vi "testMatOper.vi"(8 "error in (no error)":errorcluster) -> (0 "error out":errorcluster)   [LabVIEW 2016]
doc: "Test the MatOper class functions."
uses:
  <vilib>/addons/_JKI Toolkits/Caraya/classes/Test/Test.lvclass
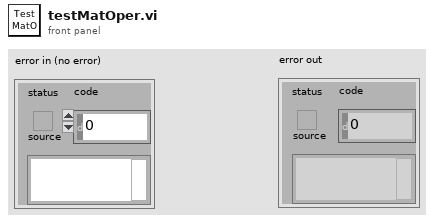
[diagram p1: front panel]
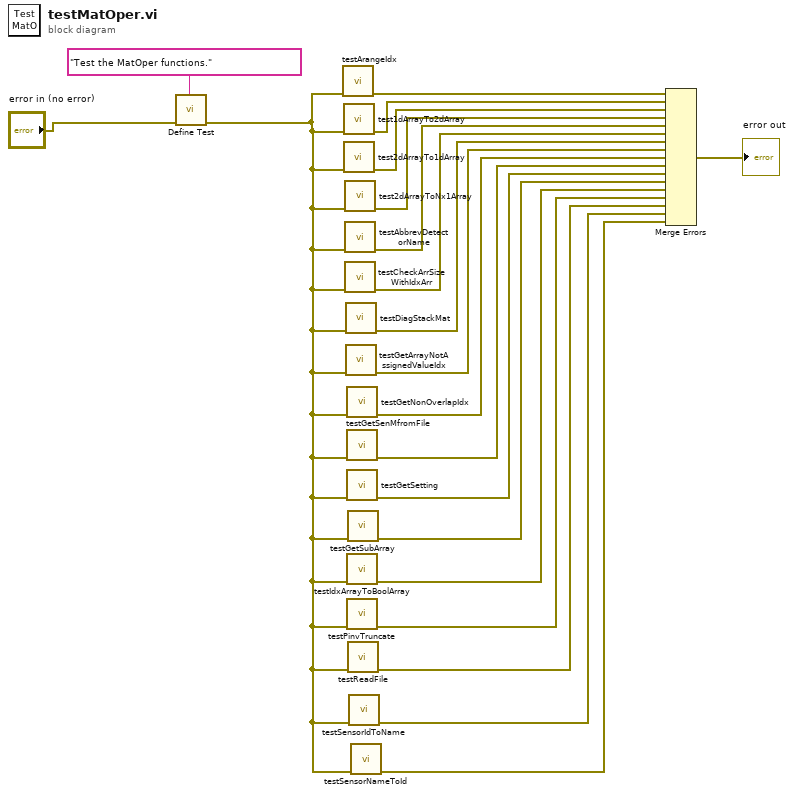
[diagram p0: block diagram]
diagram:
  n1 = call <vilib>:"Define Test.vi"("error in (no error)"="error in (no error)", "Label (VI Title)"="Test the MatOper functions.") -> ("error out"=w2:errorcluster)  [unwired: 9 in]
  n2 = call "testArangeIdx.vi"("error in (no error)"=w2) -> ("error out"=w18:errorcluster)  [unwired: 10 in]
  n3 = call "test1dArrayTo2dArray.vi"("error in (no error)"=w2) -> ("error out"=w17:errorcluster)  [unwired: 10 in]
  n4 = call "test2dArrayTo1dArray.vi"("error in (no error)"=w2) -> ("error out"=w16:errorcluster)  [unwired: 10 in]
  n5 = call "test2dArrayToNx1Array.vi"("error in (no error)"=w2) -> ("error out"=w15:errorcluster)  [unwired: 10 in]
  n6 = call "testAbbrevDetectorName.vi"("error in (no error)"=w2) -> ("error out"=w14:errorcluster)  [unwired: 10 in]
  n7 = call "testCheckArrSizeWithIdxArr.vi"("error in (no error)"=w2) -> ("error out"=w13:errorcluster)  [unwired: 10 in]
  n8 = call "testDiagStackMat.vi"("error in (no error)"=w2) -> ("error out"=w12:errorcluster)  [unwired: 10 in]
  n9 = call "testGetArrayNotAssignedValueIdx.vi"("error in (no error)"=w2) -> ("error out"=w11:errorcluster)  [unwired: 10 in]
  n10 = call "testGetNonOverlapIdx.vi"("error in (no error)"=w2) -> ("error out"=w10:errorcluster)  [unwired: 10 in]
  n11 = call "testGetSenMfromFile.vi"("error in (no error)"=w2) -> ("error out"=w9:errorcluster)  [unwired: 10 in]
  n12 = call "testGetSetting.vi"("error in (no error)"=w2) -> ("error out"=w8:errorcluster)  [unwired: 10 in]
  n13 = call "testIdxArrayToBoolArray.vi"("error in (no error)"=w2) -> ("error out"=w6:errorcluster)  [unwired: 10 in]
  n14 = call "testPinvTruncate.vi"("error in (no error)"=w2) -> ("error out"=w5:errorcluster)  [unwired: 10 in]
  n15 = call "testGetSubArray.vi"("error in (no error)"=w2) -> ("error out"=w7:errorcluster)  [unwired: 10 in]
  n16 = call "testReadFile.vi"("error in (no error)"=w2) -> ("error out"=w4:errorcluster)  [unwired: 10 in]
  n17 = call "testSensorIdToName.vi"("error in (no error)"=w2) -> ("error out"=w3:errorcluster)  [unwired: 10 in]
  n18 = call "testSensorNameToId.vi"("error in (no error)"=w2) -> ("error out"=w1:errorcluster)  [unwired: 10 in]
  n19 = Merge Errors(w18, w17, w16, w15, w14, w13, w12, w11, w10, w9, w8, w7, w6, w5, w4, w3, w1) -> (→"error out":errorcluster)
